vi "Disable Menus and Buttons.vi"(6 "menu reference in":refnum<k9>, 7 "Array":refnum<vi>[](array[refnum]), 10 "Array 3":bool[](array[boolean]), 11 "Array 2":string[](array[string])) -> ()   [LabVIEW 2015]
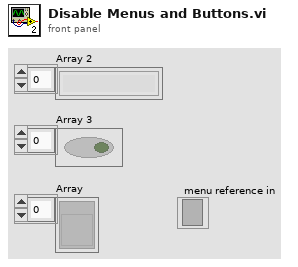
[diagram p1: front panel]
types:
  T1 = enum8{"Enabled", "Disabled", "Disabled and Grayed Out"}
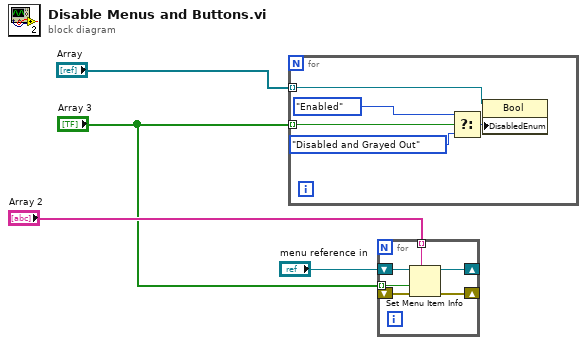
[diagram p0: block diagram]
diagram:
  n1 = for {
    tunnel: "Array" -> [w6] mode=indexing
    tunnel: "Array 3" -> [w5] mode=indexing
    n2 = Select(t=T1."Enabled" ("Disabled"), s=w5, f=T1."Disabled and Grayed Out" ("Disabled")) -> (s? t:f=w7:T1)
    n3 = property class="Bool"(reference=w6, "DisabledEnum"=w7) -> ()  [unwired: 1 in, 2 out]
  }
  n4 = for {
    shift-right: [w14] -> _
    shift-left: "menu reference in" -> [w15]
    tunnel: "Array 2" -> [w13] mode=indexing
    tunnel: "Array 3" -> [w12] mode=indexing
    shift-right: [w11] -> _
    shift-left: _ -> [w10]
    n5 = Set Menu Item Info(7:w13, 8:w10, 9:w12, 11:w15) -> (0:w11:errorcluster, 3:w14:refnum<k9>)  [unwired: 3 in]
  }
